vi "SHOOTER Vel CLOSED LOOP.vi"(0 "PhoenixMotorControlDevRef IN":T2={"DeviceStatus"={"status"=FALSE, "code"=0, "source"=""}, "Type"=enum."PWM", "PWM"={"PWM Channel"=enum."PWM 1", "DeadBand"={"Name"="", "maxPositivePwm"=0, "minPositivePwm"=0, "centerPwm"=0, "maxNegativePwm"=0, "minNegativePwm"=0, "angularRange"=0}}, "CAN"={"Device Number"=0, "SetOutput VI Ref"=variant(enum8{"Percent VBus", "Current", "Speed", "Position", "Voltage"} enum."Percent VBus"), "GetOutput VI Ref"=variant(refnum<k1> refnum), "Enable VI Ref"=variant(dbl 12.0), "Disable VI Ref"=variant(enum8{"Percent VBus", "Speed", "Position", "Slave", "Unchanged / Invalid", "Voltage Compensation", "Current", "Motion Profile"} enum."Percent VBus"), "Data"=variant}, "Invert"=FALSE, "DIO PWM"={"PWM \"Enable\" Channel"=enum."Invalid", "DIOChannel"=enum."Invalid", "PWM Rate"=0.0}}, 4 "PID Parameters":T7 {"I Zone process error" format="%.3f"; "feed-forward gain, F" format="%.5f"; "differential gain, D" min=0.0 format="%.3f"; "integral gain, I" format="%.3f"; "proportional gain, P" min=0.0 format="%.3f"}, 5 "error in (no error)":errorcluster, 6 "slotIdx":i32, 7 "arm angle table":T1) -> (14 "PhoenixMotorControlDevRef":T2={"DeviceStatus"={"status"=FALSE, "code"=0, "source"=""}, "Type"=enum."PWM", "PWM"={"PWM Channel"=enum."Invalid", "DeadBand"={"Name"="", "maxPositivePwm"=0, "minPositivePwm"=0, "centerPwm"=0, "maxNegativePwm"=0, "minNegativePwm"=0, "angularRange"=0}}, "CAN"={"Device Number"=0, "SetOutput VI Ref"=variant, "GetOutput VI Ref"=variant, "Enable VI Ref"=variant, "Disable VI Ref"=variant, "Data"=variant}, "Invert"=FALSE, "DIO PWM"={"PWM \"Enable\" Channel"=enum."Invalid", "DIOChannel"=enum."Invalid", "PWM Rate"=0.0}}, 15 "Target Velocity Units per 100ms":dbl, 19 "error out":errorcluster)   [LabVIEW 2020]
doc: "This VI is called for each TeleOp packet received from the DS where the robot is not disabled. It is often used to read from the joysticks and update I/O or to update setpoints for timed control loops. It should complete and return within 20 milliseconds or it may miss DS packets."
uses:
  <vilib>/Rock Robotics/WPI/MotorControl/WPI_MotorControlDeviceRef.ctl
  <vilib>/Rock Robotics/WPI/MotorControl/WPI_MotorControlType.ctl
  <vilib>/Rock Robotics/SystemInterfaces/DIO/FPGA_DIOPWMChannel.ctl
  <vilib>/Rock Robotics/WPI/PWM/WPI_PWMDeadband.ctl
  <vilib>/Rock Robotics/SystemInterfaces/DIO/FPGA_DIOChannel.ctl
  <vilib>/Rock Robotics/WPI/ThirdParty/Phoenix-LabVIEW/Motor Controller/Controls/CTRE_Phoenix_MotorControl_ControlMode.ctl
  <vilib>/Rock Robotics/Network Tables/NT Read Boolean.vi
  Robot Global Data.vi
  <vilib>/Rock Robotics/WPI/ThirdParty/Phoenix-LabVIEW/Motor Controller/Get/CTRE_Phoenix_MotorController_GetVoltage.vi
  <vilib>/Rock Robotics/WPI/ThirdParty/Phoenix-LabVIEW/Motor Controller/Get/CTRE_Phoenix_MotorController_IntegratedSensorData_TalonFX.vi
  <vilib>/Rock Robotics/Network Tables/NT Read Number.vi
panel:
  in  "SHOOTER control method":enum16{"Velocity PID Loop", "Percent Output"}(ring)=enum."Percent Output"
  out "motor Inverted?":bool
  out "Falcon 500 ticks/rev":i32=2048
  out "conv rpm to rad/s":dbl
  out "100% wheel speed (in/s)":dbl
  out "100% wheel speed (rad/s)":dbl
  out "wheel diameter (in)":dbl=6.0
  out "gear ratio :1":dbl=1.0
  in  "motor free (rpm)":dbl=6350.0
  in  "Overide?":bool
  in  "Throttle":dbl(knob) scale=0.0..100.0
  out "SensorPosUnits":dbl format="%.2f"
  out "Motor output Plot":cluster{"Percent Output":dbl}(graph)
  out "Sensor Velocity Units Per 100ms":dbl format="%.2f"
  out "Applied Output":dbl
  out "Speed Closed Loop Plots":cluster{dbl, "Velocity":dbl}(graph)
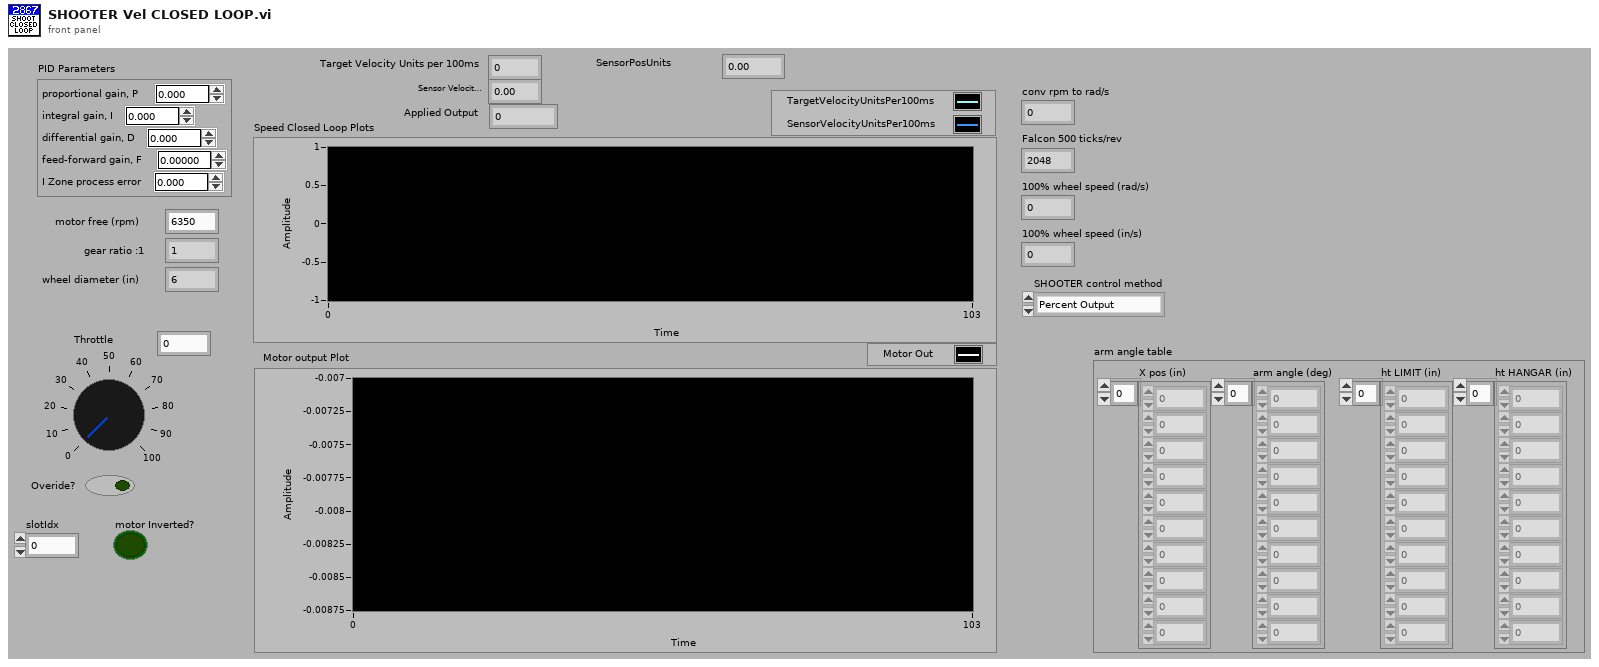
[diagram p1: front panel]
types:
  T1 = cluster{"X pos (in)":dbl[], "arm angle (deg)":dbl[], "ht LIMIT (in)":dbl[], "ht HANGAR (in)":dbl[]}
  T2 = typedef "WPI_MotorControlDeviceRef.ctl" = cluster{"DeviceStatus":errorcluster, "Type":T3, "PWM":cluster{"PWM Channel":T4, "DeadBand":T5}, "CAN":cluster{"Device Number":u8, "SetOutput VI Ref":variant, "GetOutput VI Ref":variant, "Enable VI Ref":variant, "Disable VI Ref":variant, "Data":variant}, "Invert":bool, "DIO PWM":cluster{"PWM \"Enable\" Channel":T4, "DIOChannel":T6, "PWM Rate":dbl}}
  T3 = typedef "WPI_MotorControlType.ctl" = enum16{"PWM", "CAN", "DIO PWM"}
  T4 = typedef "FPGA_DIOPWMChannel.ctl" = enum8{"PWM 0", "PWM 1", "PWM 2", "PWM 3", "PWM 4", "PWM 5", "PWM 6", "PWM 7", "PWM 8", "PWM 9", "PWM MXP 0", "PWM MXP 1", "PWM MXP 2", "PWM MXP 3", "PWM MXP 4", "PWM MXP 5", "PWM MXP 6", "PWM MXP 7", "PWM MXP 8", "PWM MXP 9", "Invalid"}
  T5 = typedef "WPI_PWMDeadband.ctl" = cluster{"Name":string, "maxPositivePwm":i32, "minPositivePwm":i32, "centerPwm":i32, "maxNegativePwm":i32, "minNegativePwm":i32, "angularRange":u16}
  T6 = typedef "FPGA_DIOChannel.ctl" = enum8{"DIO 0", "DIO 1", "DIO 2", "DIO 3", "DIO 4", "DIO 5", "DIO 6", "DIO 7", "DIO 8", "DIO 9", "DIO MXP 0", "DIO MXP 1", "DIO MXP 2", "DIO MXP 3", "DIO MXP 4", "DIO MXP 5", "DIO MXP 6", "DIO MXP 7", "DIO MXP 8", "DIO MXP 9", "DIO MXP 10", "DIO MXP 11", "DIO MXP 12", "DIO MXP 13", "DIO MXP 14", "DIO MXP 15", "SPI Port CS1", "SPI Port CS2", "SPI Port CS3", "SPI Port MISO", "SPI Port MOSI", "Invalid"}
  T7 = cluster{"proportional gain, P":dbl, "integral gain, I":dbl, "differential gain, D":dbl, "feed-forward gain, F":dbl, "I Zone process error":dbl}
  T8 = typedef "CTRE_Phoenix_MotorControl_ControlMode.ctl" = u16
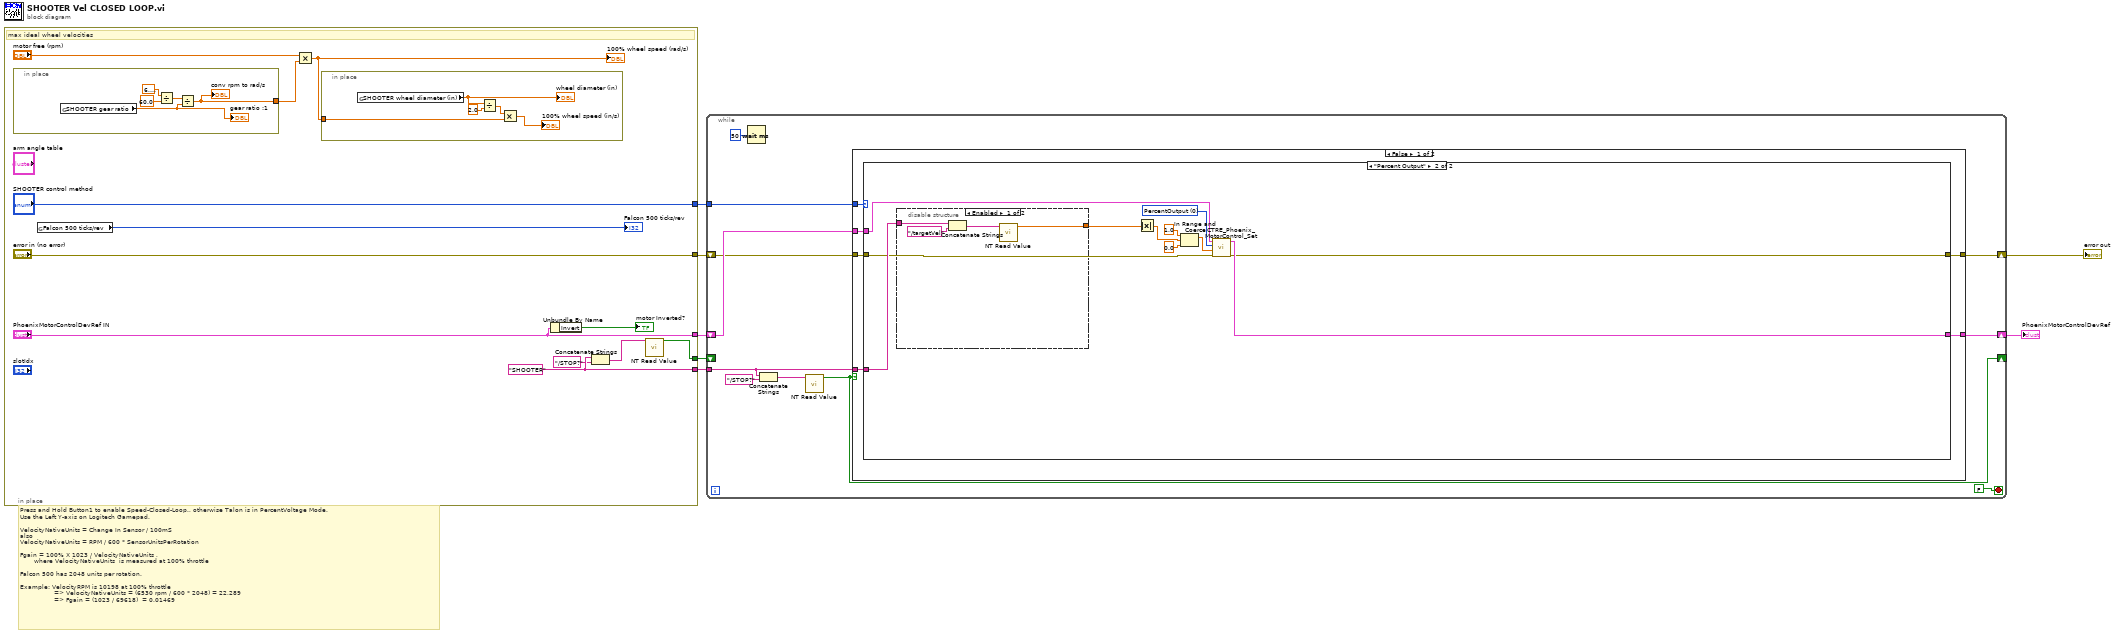
[diagram p0: block diagram]
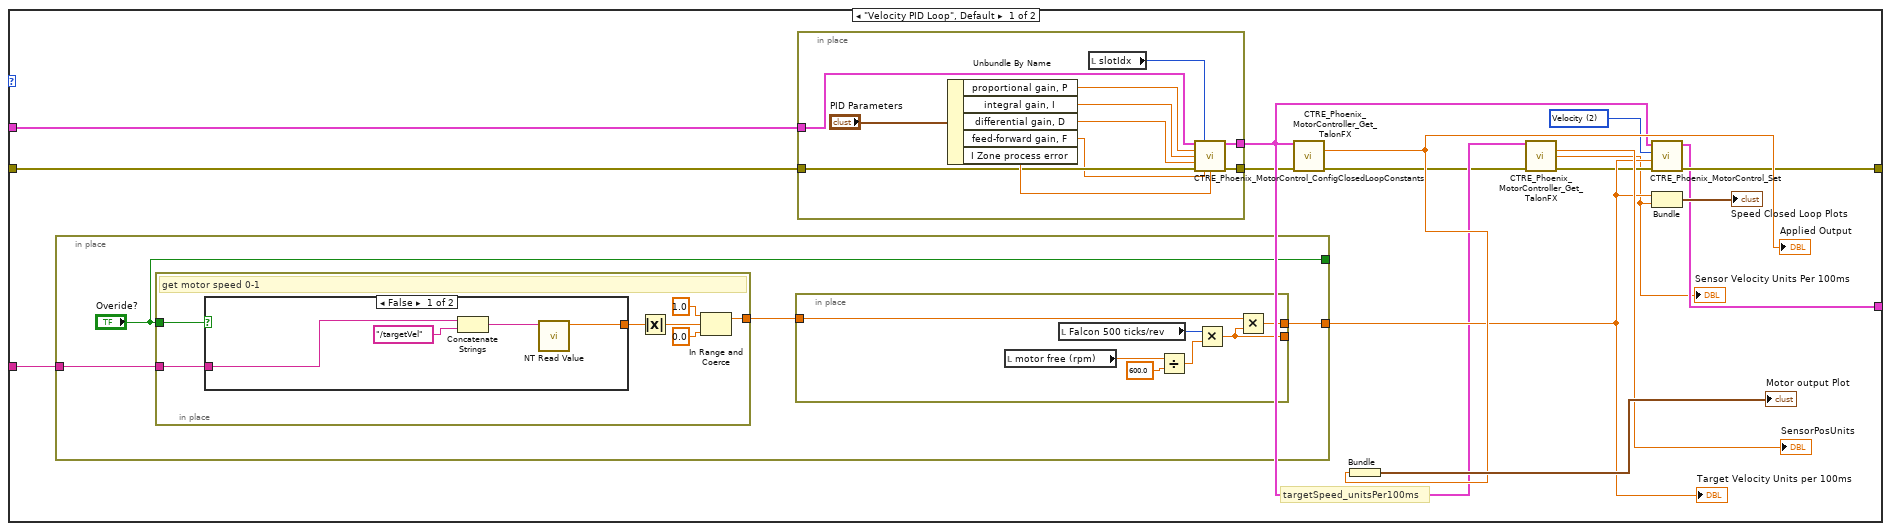
[diagram p2: hidden frame]
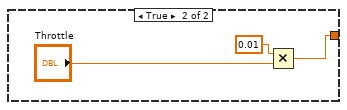
[diagram p3: hidden frame]
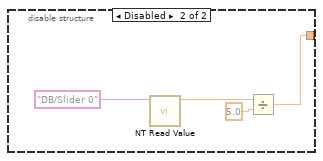
[diagram p4: hidden frame]
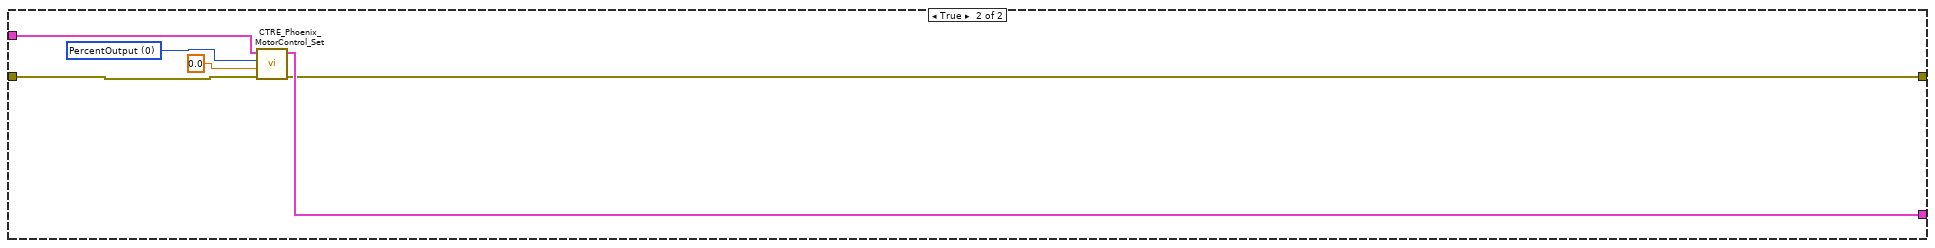
[diagram p5: hidden frame]
diagram:
  # "Press and Hold Button1 to enable Speed-Closed-Loop., otherwise Talon is in PercentVoltage Mode.  \nUse the Left Y-axis on Logitech Gamepad.\n\nVelocityNativeUnits = Change In Sensor / 100mS\nalso\nVelocityNativeUnits = RPM / 600 * SensorUnitsPerRotation\n\nFgain = 100% X 1023 / VelocityNativeUnits , \n       where VelocityNativeUnits  is measured at 100% throttle\n\nFalcon 500 has 2048 units per rotation.\n\nExample: VelocityRPM is 10198 at 100% throttle\n                 => VelocityNativeUnits = (6530 rpm / 600 * 2048) = 22,289\n                 => Fgain = (1023 / 69618)  = 0.01469"
  n1 = in-place {
    in-place-border: ["PhoenixMotorControlDevRef IN"] -> w7
    in-place-border: [w14] -> w6
    in-place-border: [w11] -> w3
    in-place-border: ["error in (no error)"] -> w5
    in-place-border: ["SHOOTER control method"] -> w4
    w14 = "SHOOTER"
    # "max ideal wheel velocities"
    n2 = in-place {
      in-place-border: [w21] -> w19
      n3 = global read "Robot Global Data.vi" "SHOOTER gear ratio"() -> (w20:dbl)
      "gear ratio :1" <- w20
      n4 = Divide(x=6.283185307179586, y=60.0) -> (x/y=w22:dbl)
      n5 = Divide(x=w22, y=w20) -> (x/y=w21:dbl)
      "conv rpm to rad/s" <- w21
    }
    n6 = global read "Robot Global Data.vi" "Falcon 500 ticks/rev"() -> (→"Falcon 500 ticks/rev":i32)
    n7 = Multiply(x="motor free (rpm)", y=w19) -> (x*y=w17:dbl)
    "100% wheel speed (rad/s)" <- w17
    n8 = in-place {
      in-place-border: w17 -> [w27]
      n9 = global read "Robot Global Data.vi" "SHOOTER wheel diameter (in)"() -> (w25:dbl)
      "wheel diameter (in)" <- w25
      n10 = Divide(x=w25, y=2.0) -> (x/y=w28:dbl)
      n11 = Multiply(x=w28, y=w27) -> (x*y=→"100% wheel speed (in/s)":dbl)
    }
    n12 = Unbundle By Name("PhoenixMotorControlDevRef IN") -> ("Invert"=→"motor Inverted?":bool)
    n13 = Concatenate Strings(w14, "/STOP?" ("string")) -> (w13:string)
    n14 = call-poly <vilib>:"NT Read Value.vi"("Name"=w13) -> ("Boolean"=w11:bool)  [unwired: 9 in, 1 out]
  }
  n15 = while {
    tunnel: w6 -> [w37]
    tunnel: w4 -> [w38]
    shift-right: [w35] -> _
    shift-left: w3 -> [_]
    shift-right: [w34] -> w2
    shift-left: w7 -> [w40]
    shift-right: [w31] -> w1
    shift-left: w5 -> [w39]
    stop <- FALSE stop-if-true
    n16 = Wait (ms)(milliseconds to wait=u32 50) -> ()  [unwired: 1 out]
    n17 = Concatenate Strings(w37, "/STOP?" ("string")) -> (w32:string)
    n18 = call-poly <vilib>:"NT Read Value.vi"("Name"=w32) -> ("Boolean"=w35:bool)  [unwired: 9 in, 1 out]
    n19 = case shown="False" w35 {
      tunnel: w40 -> [w46 w123]
      tunnel: [w45 w118] -> w31
      tunnel: [w44 w120] -> w34
      tunnel: w39 -> [w43 w119]
      tunnel: w38 -> [w42 _]
      tunnel: w37 -> [w41 _]
      frame False {
        n20 = case shown="\"Percent Output\"" w42 {
          tunnel: w41 -> [w57 w109]
          tunnel: w46 -> [w56 w106]
          tunnel: [w53 w103] -> w45
          tunnel: [w52 w104] -> w44
          tunnel: w43 -> [w51 w105]
          frame "Velocity PID Loop", Default {
            w54 = T8 2 items=["PercentOutput"=0, "Position"=1, "Velocity"=2, "Follower"=5, "MotionProfile"=6, "MotionMagic"=7, "MotionMagicArc"=8, "TimedPercentOutput"=9, "Disabled"=15] ("Control Mode")
            # "targetSpeed_unitsPer100ms"
            n21 = in-place {
              in-place-border: [w75] -> w58
              in-place-border: w57 -> [w77]
              in-place-border: ["Overide?"] -> _
              n22 = in-place {
                in-place-border: w77 -> [w84]
                in-place-border: "Overide?" -> [w83]
                in-place-border: [w80] -> w74
                # "get motor speed 0-1"
                n23 = case shown="False" w83 {
                  tunnel: [w85 w89] -> w82
                  tunnel: w84 -> [w87 _]
                  frame False {
                    n24 = Concatenate Strings(w87, "/targetVel" ("string")) -> (w88:string)
                    n25 = call-poly <vilib>:"NT Read Value.vi"("Name"=w88) -> ("Numeric"=w85:dbl)  [unwired: 9 in, 1 out]
                  }
                  frame True {
                    n26 = Multiply(x=0.01, y="Throttle") -> (x*y=w89:dbl)
                  }
                }
                n27 = Absolute Value(x=w82) -> (abs(x)=w81:dbl)
                n28 = In Range and Coerce(upper limit=1.0, x=w81, lower limit=0.0 ("upper limit")) -> (coerced(x)=w80:dbl)  [unwired: 1 out]
              }
              n29 = in-place {
                in-place-border: w74 -> [w93]
                in-place-border: [w94] -> w75
                in-place-border: [w92] -> _
                n30 = local read "motor free (rpm)"() -> (w95:dbl)
                n31 = local read "Falcon 500 ticks/rev"() -> (w98:i32)
                n32 = Divide(x=w95, y=600.0) -> (x/y=w97:dbl)
                n33 = Multiply(x=w98, y=w97) -> (x*y=w92:dbl)
                n34 = Multiply(x=w93, y=w92) -> (x*y=w94:dbl)
              }
            }
            "Target Velocity Units per 100ms" <- w58
            n35 = in-place {
              in-place-border: [w73] -> w55
              in-place-border: w56 -> [w67]
              in-place-border: w51 -> [w65]
              in-place-border: [w64] -> w50
              n36 = Unbundle By Name("PID Parameters") -> ("proportional gain, P"=w71:dbl, "integral gain, I"=w70:dbl, "differential gain, D"=w69:dbl, "feed-forward gain, F"=w63:dbl, "I Zone process error"=w68:dbl)
              n37 = local read "slotIdx"() -> (w66:i32)
              n38 = call <vilib>:"CTRE_Phoenix_MotorControl_ConfigClosedLoopConstants.vi"("PhoenixMotorControlDevRef"=w67, "slotIdx"=w66, "P"=w71, "I"=w70, "D"=w69, "error in (no error)"=w65, "F"=w63, "I Zone"=w68) -> ("PhoenixMotorControlDevRef"=w73:T2, "error out"=w64:errorcluster)  [unwired: 6 in]
            }
            n39 = call-poly <vilib>:"CTRE_Phoenix_MotorController_Get_TalonFX.vi"("PhoenixMotorControlDevRef"=w55, "error in"=w50) -> ("Percent Output"=w59:dbl, "error out"=w49:errorcluster)  [unwired: 9 in, 3 out]
            "Applied Output" <- w59
            n40 = Bundle("Percent Output"=w59) -> (→"Motor output Plot":cluster{"Percent Output":dbl})  [unwired: 1 in]
            n41 = call-poly <vilib>:"CTRE_Phoenix_MotorController_Get_TalonFX.vi"("PhoenixMotorControlDevRef"=w55, "error in"=w49) -> ("Position"=→"SensorPosUnits":dbl, "Velocity"=w47:dbl, "error out"=w48:errorcluster)  [unwired: 9 in, 2 out]
            "Sensor Velocity Units Per 100ms" <- w47
            n42 = call <vilib>:"CTRE_Phoenix_MotorControl_Set.vi"("error in (no error)"=w48, "Output"=w58, "Control Mode"=w54, "PhoenixMotorControlDevRef"=w55) -> ("error out"=w53:errorcluster, "PhoenixMotorControlDevRef"=w52:T2)  [unwired: 6 in]
            n43 = Bundle(w58, "Velocity"=w47) -> (→"Speed Closed Loop Plots":cluster{dbl, "Velocity":dbl})  [unwired: 1 in]
          }
          frame "Percent Output" {
            w108 = T8 0 items=["PercentOutput"=0, "Position"=1, "Velocity"=2, "Current"=3, "Follower"=5, "MotionProfile"=6, "MotionMagic"=7, "MotionProfileArc"=10, "Disabled"=15] ("Control Mode")
            n44 = disable-structure shown="Enabled" {
              disable-tunnel: w109 -> [w111 _]
              disable-tunnel: [w110 w115] -> w107
              frame Enabled {
                n45 = Concatenate Strings(w111, "/targetVel" ("string")) -> (w112:string)
                n46 = call-poly <vilib>:"NT Read Value.vi"("Name"=w112) -> ("Numeric"=w110:dbl)  [unwired: 9 in, 1 out]
              }
              frame Disabled {
                n47 = call-poly <vilib>:"NT Read Value.vi"("Name"="DB/Slider 0") -> ("Numeric"=w116:dbl)  [unwired: 9 in, 1 out]
                n48 = Divide(x=w116, y=5.0) -> (x/y=w115:dbl)
              }
            }
            n49 = Absolute Value(x=w107) -> (abs(x)=w99:dbl)
            n50 = In Range and Coerce(upper limit=1.0, x=w99, lower limit=0.0) -> (coerced(x)=w102:dbl)  [unwired: 1 out]
            n51 = call <vilib>:"CTRE_Phoenix_MotorControl_Set.vi"("error in (no error)"=w105, "Output"=w102, "Control Mode"=w108, "PhoenixMotorControlDevRef"=w106) -> ("error out"=w103:errorcluster, "PhoenixMotorControlDevRef"=w104:T2)  [unwired: 6 in]
          }
        }
      }
      frame True {
        w122 = T8 0 items=["PercentOutput"=0, "Position"=1, "Velocity"=2, "Current"=3, "Follower"=5, "MotionProfile"=6, "MotionMagic"=7, "MotionProfileArc"=10, "Disabled"=15] ("Control Mode")
        n52 = call <vilib>:"CTRE_Phoenix_MotorControl_Set.vi"("error in (no error)"=w119, "Output"=0.0, "Control Mode"=w122, "PhoenixMotorControlDevRef"=w123) -> ("error out"=w118:errorcluster, "PhoenixMotorControlDevRef"=w120:T2)  [unwired: 6 in]
      }
    }
  }
  "error out" <- w1
  "PhoenixMotorControlDevRef" <- w2
